vi "Read Controllers.vi"   [LabVIEW 2014]
uses:
  Begin/Global RefNums.vi
  <vilib>/Rock Robotics/WPI/Joystick/WPI_JoystickGetSetRefNum.vi
  Begin/Global Variables.vi
types:
  T1 = typedef "WPI_JoystickDevRef.ctl" = cluster{"Device":T2}
  T2 = typedef "WPI_JoystickDeviceEnum.ctl" = enum16{"USB 0", "USB 1", "USB 2", "USB 3", "USB 4", "USB 5"}
  T3 = cluster{"Buttons[0]":bool, "Buttons[1]":bool, "Buttons[2]":bool, "Buttons[3]":bool, "Buttons[4]":bool, "Buttons[5]":bool, "Buttons[6]":bool, "Buttons[7]":bool, "Buttons[8]":bool}
  T4 = cluster{"Axes[0]":dbl, "Axes[1]":dbl, "Axes[2]":dbl, "Axes[3]":dbl, "Axes[4]":dbl, "Axes[5]":dbl, "Axes[6]":dbl, "Axes[7]":dbl, "Axes[8]":dbl}
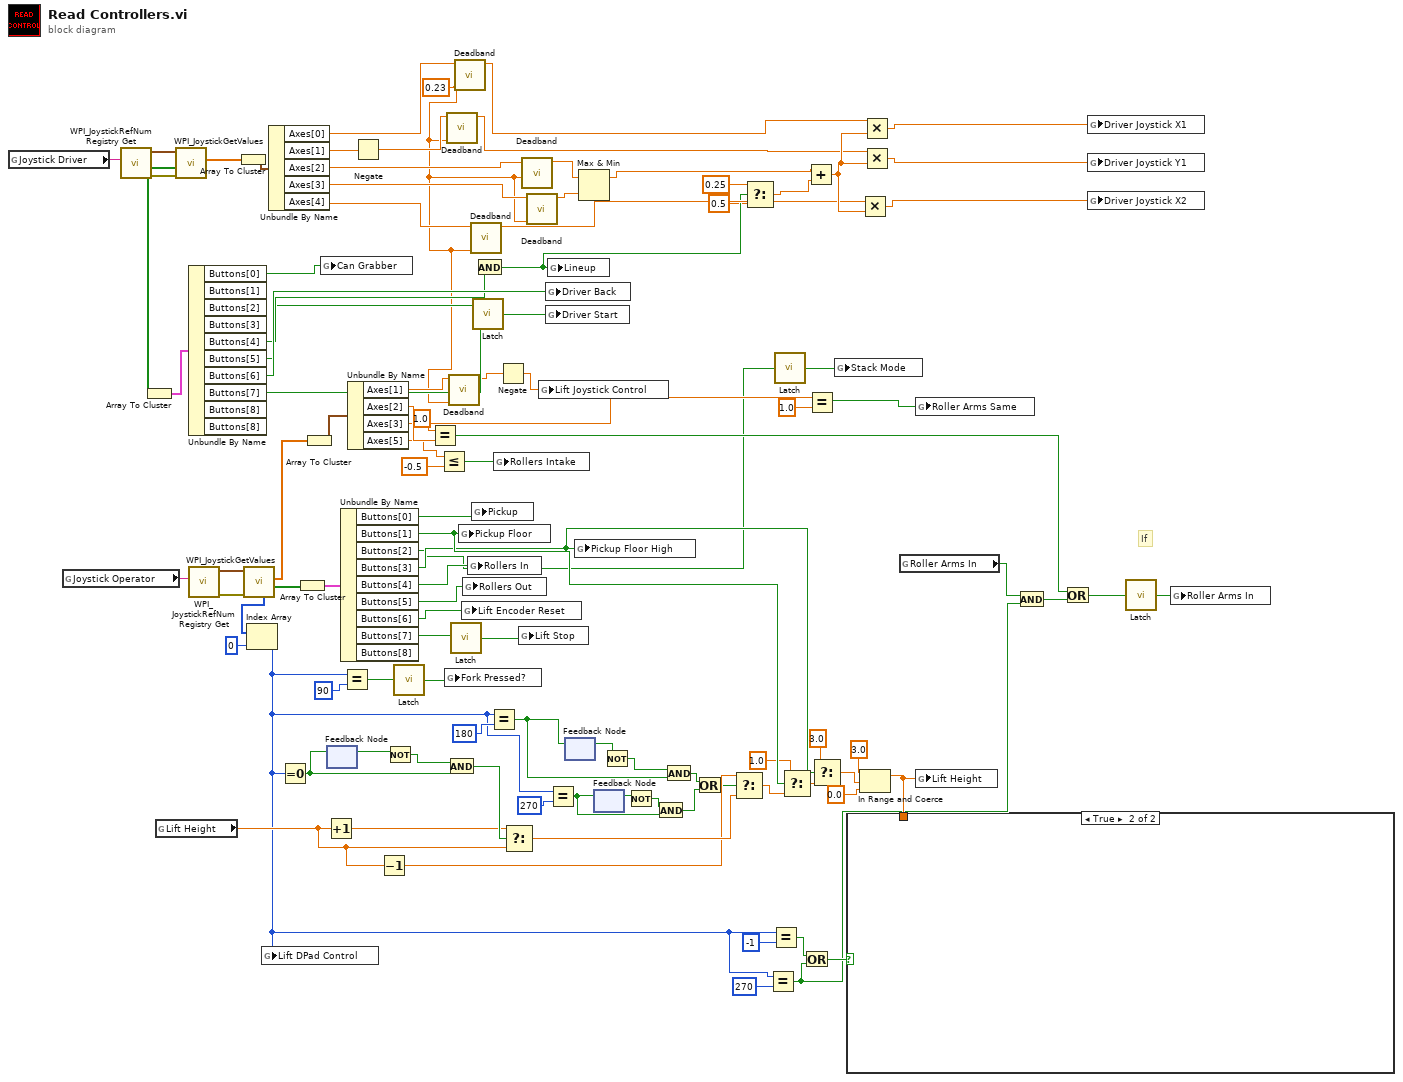
[diagram p0: block diagram]
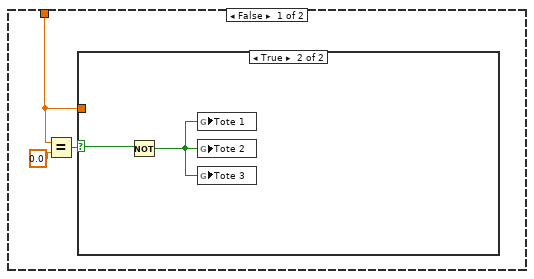
[diagram p2: hidden frame]
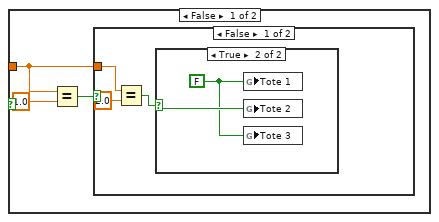
[diagram p3: hidden frame]
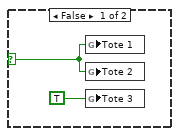
[diagram p4: hidden frame]
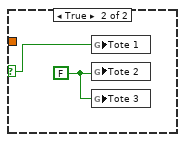
[diagram p5: hidden frame]
diagram:
  w24 = 0.23 ("Value to Deadband (default of 0.1)")
  # "If"
  n1 = global read "Global RefNums.vi" "Joystick Driver"() -> (w105:string)
  n2 = global read "Global RefNums.vi" "Joystick Operator"() -> (w100:string)
  n3 = call <vilib>:"WPI_JoystickRefNum Registry Get.vi"("refnum name"=w105) -> ("error out"=w103:errorcluster, "JoystickDevRef"=w104:T1)  [unwired: 9 in]
  n4 = global read "Global Variables.vi" "Lift Height"() -> (w77:dbl)
  n5 = call <vilib>:"WPI_JoystickGetValues.vi"("error in (no error)"=w103, "JoystickDevRef"=w104) -> ("Buttons"=w97:bool[], "Axes"=w99:dbl[])  [unwired: 5 in, 3 out]
  n6 = Array To Cluster(array=w97) -> (cluster=w96:T3)
  n7 = Unbundle By Name(w96) -> ("Buttons[0]"=w27:bool, "Buttons[4]"=w44:bool, "Buttons[5]"=w43:bool, "Buttons[6]"=w71:bool, "Buttons[7]"=w73:bool)  [unwired: 5 out]
  n8 = call <vilib>:"WPI_JoystickRefNum Registry Get.vi"("refnum name"=w100) -> ("error out"=w102:errorcluster, "JoystickDevRef"=w101:T1)  [unwired: 9 in]
  n9 = Array To Cluster(array=w99) -> (cluster=w98:T4)
  n10 = call <vilib>:"WPI_JoystickGetValues.vi"("error in (no error)"=w102, "JoystickDevRef"=w101) -> ("Buttons"=w94:bool[], "Axes"=w69:dbl[], "POVs"=w89:i16[])  [unwired: 5 in, 2 out]
  n11 = Index Array(array=w89, index=0) -> (element=w36:i16)
  n12 = global write "Global Variables.vi" "Lift DPad Control"(w36) -> ()
  n13 = Unbundle By Name(w98) -> ("Axes[0]"=w95:dbl, "Axes[1]"=w56:dbl, "Axes[2]"=w26:dbl, "Axes[3]"=w25:dbl, "Axes[4]"=w57:dbl)
  n14 = Equal To 0?(x=w36) -> (x = 0?=w85:bool)
  n15 = Array To Cluster(array=w94) -> (cluster=w93:T3)
  n16 = Array To Cluster(array=w69) -> (cluster=w68:T4)
  n17 = global write "Global Variables.vi" "Can Grabber"(w27) -> ()
  n18 = Increment(x=w77) -> (x+1=w83:dbl)
  n19 = feedback-in #1(w85) -> ()
  n20 = feedback #1() -> (w87:bool)  [unwired: 1 in]
  n21 = Unbundle By Name(w93) -> ("Buttons[0]"=w92:bool, "Buttons[1]"=w33:bool, "Buttons[2]"=w1:bool, "Buttons[3]"=w30:bool, "Buttons[4]"=w67:bool, "Buttons[5]"=w66:bool, "Buttons[6]"=w65:bool, "Buttons[7]"=w91:bool)  [unwired: 1 out]
  n22 = Equal?(x=w36, y=i16 90) -> (x = y?=w53:bool)
  n23 = Unbundle By Name(w68) -> ("Axes[1]"=w64:dbl, "Axes[2]"=w58:dbl, "Axes[3]"=w5:dbl, "Axes[5]"=w6:dbl)
  n24 = Negate(x=w56) -> (-x=w55:dbl)
  n25 = Decrement(x=w77) -> (x-1=w76:dbl)
  n26 = Not(x=w87) -> (.not. x?=w86:bool)
  n27 = call "Latch.vi"("Input"=w53) -> ("Output"=w52:bool)
  n28 = Equal?(x=1.0, y=w58) -> (x = y?=w48:bool)
  n29 = Less Or Equal?(x=w6, y=-0.5) -> (x <= y?=w7:bool)
  n30 = global write "Global Variables.vi" "Fork Pressed?"(w52) -> ()
  n31 = call "Deadband.vi"("Value to Deadband (default of 0.1)"=w24, "Value"=w55) -> ("Deadbanded Value"=w18:dbl)  [unwired: 9 in]
  n32 = And(x=w86, y=w85) -> (x .and. y?=w84:bool)
  n33 = call "Deadband.vi"("Value to Deadband (default of 0.1)"=w24, "Value"=w64) -> ("Deadbanded Value"=w62:dbl)  [unwired: 9 in]
  n34 = call "Latch.vi"("Input"=w91) -> ("Output"=w90:bool)
  n35 = call "Deadband.vi"("Value to Deadband (default of 0.1)"=w24, "Value"=w95) -> ("Deadbanded Value"=w19:dbl)  [unwired: 9 in]
  n36 = global write "Global Variables.vi" "Pickup Floor"(w33) -> ()
  n37 = global write "Global Variables.vi" "Lift Encoder Reset"(w65) -> ()
  n38 = global write "Global Variables.vi" "Rollers Out"(w66) -> ()
  n39 = global write "Global Variables.vi" "Rollers In"(w67) -> ()
  n40 = call "Deadband.vi"("Value to Deadband (default of 0.1)"=w24, "Value"=w57) -> ("Deadbanded Value"=w17:dbl)  [unwired: 9 in]
  n41 = global write "Global Variables.vi" "Pickup"(w92) -> ()
  n42 = call "Latch.vi"("Input"=w73) -> ("Output"=w72:bool)
  n43 = And(x=w44, y=w43) -> (x .and. y?=w14:bool)
  n44 = Equal?(x=w36, y=i16 180) -> (x = y?=w81:bool)
  n45 = global write "Global Variables.vi" "Rollers Intake"(w7) -> ()
  n46 = Negate(x=w62) -> (-x=w61:dbl)
  n47 = Select(t=w83, s=w84, f=w77) -> (s? t:f=w78:dbl)
  n48 = global write "Global Variables.vi" "Lift Stop"(w90) -> ()
  n49 = call "Deadband.vi"("Value to Deadband (default of 0.1)"=w24, "Value"=w26) -> ("Deadbanded Value"=w22:dbl)  [unwired: 9 in]
  n50 = call "Deadband.vi"("Value to Deadband (default of 0.1)"=w24, "Value"=w25) -> ("Deadbanded Value"=w23:dbl)  [unwired: 9 in]
  n51 = global write "Global Variables.vi" "Lift Joystick Control"(w61) -> ()
  n52 = global write "Global Variables.vi" "Driver Back"(w71) -> ()
  n53 = global write "Global Variables.vi" "Driver Start"(w72) -> ()
  n54 = global write "Global Variables.vi" "Lineup"(w14) -> ()
  n55 = Equal?(x=w36, y=i16 270) -> (x = y?=w42:bool)
  n56 = feedback #2() -> (w80:bool)  [unwired: 1 in]
  n57 = feedback-in #2(w81) -> ()
  n58 = global write "Global Variables.vi" "Pickup Floor High"(w30) -> ()
  n59 = Max & Min(x=w22, y=w23) -> (max(x,y)=w21:dbl)  [unwired: 1 out]
  n60 = feedback #3() -> (w40:bool)  [unwired: 1 in]
  n61 = feedback-in #3(w42) -> ()
  n62 = Not(x=w80) -> (.not. x?=w79:bool)
  n63 = Not(x=w40) -> (.not. x?=w41:bool)
  n64 = And(x=w41, y=w42) -> (x .and. y?=w38:bool)
  n65 = And(x=w79, y=w81) -> (x .and. y?=w39:bool)
  n66 = Or(x=w39, y=w38) -> (x .or. y?=w37:bool)
  n67 = Select(t=w76, s=w37, f=w78) -> (s? t:f=w34:dbl)
  n68 = Select(t=0.25, s=w14, f=0.5) -> (s? t:f=w12:dbl)
  n69 = Equal?(x=w36, y=i16 270) -> (x = y?=w49:bool)
  n70 = Equal?(x=w36, y=i16 -1) -> (x = y?=w60:bool)
  n71 = call "Latch.vi"("Input"=w1) -> ("Output"=w2:bool)
  n72 = Select(t=1.0, s=w33, f=w34) -> (s? t:f=w31:dbl)
  n73 = Or(x=w60, y=w49) -> (x .or. y?=w51:bool)
  n74 = Add(x=w21, y=w12) -> (x+y=w20:dbl)
  n75 = Equal?(x=w5, y=1.0) -> (x = y?=w3:bool)
  n76 = Select(t=3.0, s=w30, f=w31) -> (s? t:f=w28:dbl)
  n77 = global write "Global Variables.vi" "Stack Mode"(w2) -> ()
  n78 = Multiply(x=w17, y=w20) -> (x*y=w16:dbl)
  n79 = In Range and Coerce(upper limit=3.0, x=w28, lower limit=0.0) -> (coerced(x)=w70:dbl)  [unwired: 1 out]
  n80 = case shown="True" w51 {
    tunnel: w70 -> [w108 _]
    frame False {
      n81 = Equal?(x=w108, y=0.0) -> (x = y?=w107:bool)
      n82 = case shown="True" w107 {
        selector: w107 -> [_ w122]
        tunnel: w108 -> [w109 _]
        frame False {
          n83 = Equal?(x=w109, y=1.0) -> (x = y?=w110:bool)
          n84 = case shown="False" w110 {
            selector: w110 -> [_ w119]
            tunnel: w109 -> [w114 _]
            frame False {
              n85 = Equal?(x=w114, y=2.0) -> (x = y?=w112:bool)
              n86 = case shown="True" w112 {
                selector: w112 -> [w115 w118]
                frame False {
                  n87 = global write "Global Variables.vi" "Tote 1"(w115) -> ()
                  n88 = global write "Global Variables.vi" "Tote 2"(w115) -> ()
                  n89 = global write "Global Variables.vi" "Tote 3"(TRUE ("Tote 2")) -> ()
                }
                frame True {
                  w117 = FALSE ("Tote 0")
                  n90 = global write "Global Variables.vi" "Tote 1"(w117) -> ()
                  n91 = global write "Global Variables.vi" "Tote 2"(w118) -> ()
                  n92 = global write "Global Variables.vi" "Tote 3"(w117) -> ()
                }
              }
            }
            frame True {
              w120 = FALSE ("Tote 1")
              n93 = global write "Global Variables.vi" "Tote 1"(w119) -> ()
              n94 = global write "Global Variables.vi" "Tote 2"(w120) -> ()
              n95 = global write "Global Variables.vi" "Tote 3"(w120) -> ()
            }
          }
        }
        frame True {
          n96 = Not(x=w122) -> (.not. x?=w121:bool)
          n97 = global write "Global Variables.vi" "Tote 1"(w121) -> ()
          n98 = global write "Global Variables.vi" "Tote 2"(w121) -> ()
          n99 = global write "Global Variables.vi" "Tote 3"(w121) -> ()
        }
      }
    }
    frame True {
    }
  }
  n100 = Multiply(x=w19, y=w20) -> (x*y=w10:dbl)
  n101 = Multiply(x=w18, y=w20) -> (x*y=w15:dbl)
  n102 = global read "Global Variables.vi" "Roller Arms In"() -> (w50:bool)
  n103 = global write "Global Variables.vi" "Roller Arms Same"(w3) -> ()
  n104 = global write "Global Variables.vi" "Lift Height"(w70) -> ()
  n105 = And(x=w50, y=w49) -> (x .and. y?=w47:bool)
  n106 = Or(x=w48, y=w47) -> (x .or. y?=w46:bool)
  n107 = global write "Global Variables.vi" "Driver Joystick X1"(w10) -> ()
  n108 = global write "Global Variables.vi" "Driver Joystick Y1"(w15) -> ()
  n109 = global write "Global Variables.vi" "Driver Joystick X2"(w16) -> ()
  n110 = call "Latch.vi"("Input"=w46) -> ("Output"=w45:bool)
  n111 = global write "Global Variables.vi" "Roller Arms In"(w45) -> ()
